vi "mcc_etc_DIO_close.vi"(8 "error in":errorcluster, 10 "input_line":refnum<k24>, 11 "output_line":refnum<k24>) -> (0 "error out":errorcluster)   [LabVIEW 2019]
uses:
  C:/Program Files (x86)/National Instruments/LabVIEW 2019/vi.lib/ULx/ULx_LV.dll
  Program Files (x86)/National Instruments/LabVIEW 2019/vi.lib/ULx/ULx_LV.dll
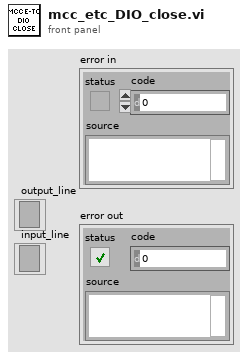
[diagram p1: front panel]
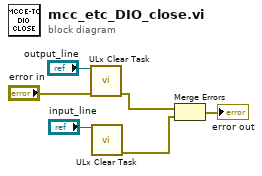
[diagram p0: block diagram]
diagram:
  n1 = call <vilib>:"ULx Clear Task.vi"("task in"="output_line", "error in"="error in") -> ("error out"=w4:errorcluster)  [unwired: 13 in]
  n2 = call <vilib>:"ULx Clear Task.vi"("task in"="input_line") -> ("error out"=w3:errorcluster)  [unwired: 14 in]
  n3 = Merge Errors(w4, w3) -> (→"error out":errorcluster)
